vi "Configure Offset Angle.vi"(8 "error in (no error)":errorcluster, 10 "ccw offset angle (rad)":dbl, 11 "NI_Robotics_Starter Kit Servo Motor_1.0 in":refnum<class "NI_Robotics_Starter Kit Servo Motor_1.0.lvclass">) -> (0 "error out":errorcluster, 3 "NI_Robotics_Starter Kit Servo Motor_1.0 out":refnum<class "NI_Robotics_Starter Kit Servo Motor_1.0.lvclass">)   [LabVIEW 2017, in "NI_Robotics_Starter Kit Servo Motor_1.0.lvclass"]
uses:
  <vilib>/robotics/Starter Kit/Servo Motor 1.0/NI_Robotics_Starter Kit Servo Motor_1.0.lvclass
  <vilib>/robotics/Starter Kit/Servo Motor 1.0/NI_Robotics_Starter Kit Servo Motor_1.0.lvclass/NI_Robotics_Starter Kit Servo Motor_1.0.ctl
  <instrlib>/Parallax Standard Servo/HAIOL/Parallax Standard Servo.lvclass
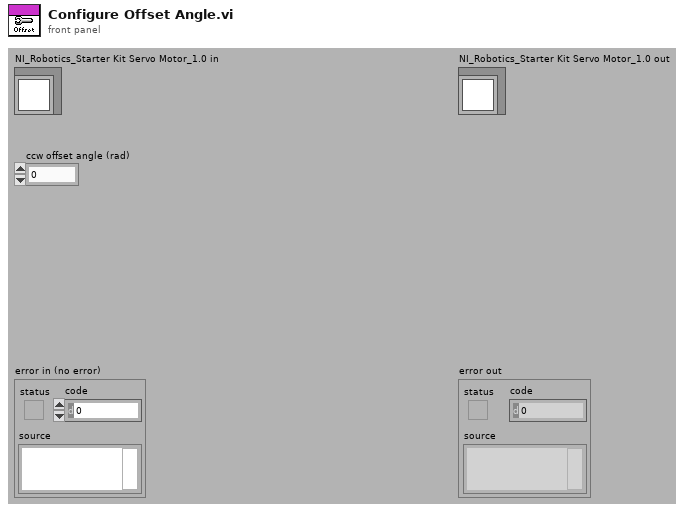
[diagram p1: front panel]
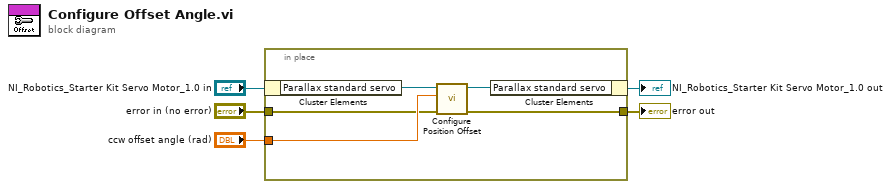
[diagram p0: block diagram]
diagram:
  n1 = in-place {
    in-place-border: "ccw offset angle (rad)" -> [w8]
    in-place-border: "error in (no error)" -> [w7]
    in-place-border: [w6] -> w1
    n2 = in-place-cluster #1("NI_Robotics_Starter Kit Servo Motor_1.0 in") -> ("Parallax standard servo"=w10:refnum<class "Parallax Standard Servo.lvclass">)
    n3 = call-dynamic "Configure Position Offset.vi"("error in (no error)"=w7, "CCW Position Offset (0.0 rad)"=w8, "Parallax Standard Servo in"=w10) -> ("error out"=w6:errorcluster, "Parallax Standard Servo out"=w9:refnum<class "Parallax Standard Servo.lvclass">)  [unwired: 7 in]
    n4 = in-place-cluster #1("Parallax standard servo"=w9) -> (→"NI_Robotics_Starter Kit Servo Motor_1.0 out":refnum<class "NI_Robotics_Starter Kit Servo Motor_1.0.lvclass">)
  }
  "error out" <- w1
